vi "SRV_VIG_QR.vi"(7 "QR Code":string, 9 "Images Directory Path":path, 12 "Method (Get and Reset)":enum16{"Get and Reset", "Set"}(ring)) -> (4 "QR?":bool, 6 "Timestamp String out":string, 8 "QR Code out":string, 10 "Images Directory Path out":path)   [LabVIEW 2014]
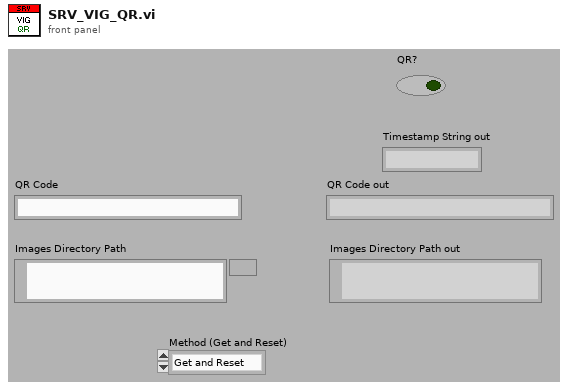
[diagram p1: front panel]
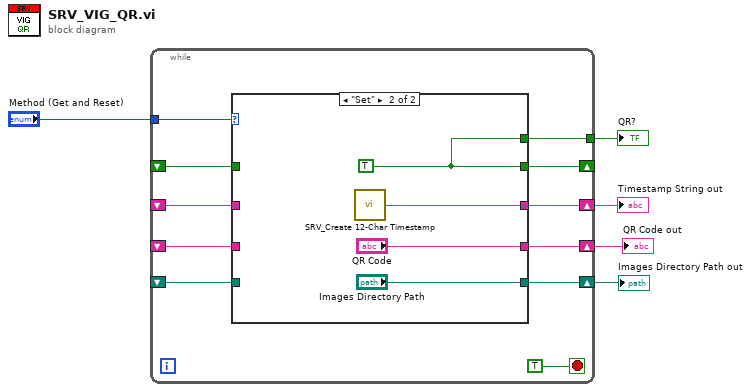
[diagram p0: block diagram]
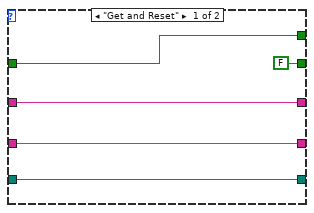
[diagram p2: hidden frame]
diagram:
  n1 = while {
    tunnel: "Method (Get and Reset)" -> [w16]
    shift-right: [w14] -> _
    shift-left: _ -> [w15]
    shift-right: [w12] -> w5
    shift-left: _ -> [w11]
    shift-right: [w10] -> w4
    shift-left: _ -> [w9]
    tunnel: [w8] -> w2
    shift-right: [w6] -> w1
    shift-left: _ -> [w7]
    stop <- TRUE stop-if-true
    n2 = case shown="\"Set\"" w16 {
      tunnel: w15 -> [w19 _]
      tunnel: [FALSE ("Movie?") w23] -> w14
      tunnel: [w21 w25] -> w12
      tunnel: w11 -> [w21 _]
      tunnel: [w20 "Images Directory Path"] -> w10
      tunnel: w9 -> [w20 _]
      tunnel: [w19 w23] -> w8
      tunnel: w7 -> [w17 _]
      tunnel: [w17 "QR Code"] -> w6
      frame "Get and Reset" {
      }
      frame "Set" {
        w23 = TRUE ("Movie?")
        n3 = call "SRV_Create 12-Char Timestamp.vi"() -> ("Timestamp String"=w25:string)  [unwired: 15 in]
      }
    }
  }
  "QR?" <- w2
  "Timestamp String out" <- w5
  "Images Directory Path out" <- w4
  "QR Code out" <- w1
